vi "DBSCAN.vi"(8 "error in":errorcluster) -> (0 "error out":errorcluster, 3 "out":refnum<class "DBSCAN.lvclass">)   [LabVIEW 2020]
doc: "Perform DBSCAN clustering from vector array or distance matrix.\n\n DBSCAN - Density-Based Spatial Clustering of Applications with Noise.\n Finds core samples of high density and expands clusters from them.\n Good for data which contains clusters of similar density.\n\n Read more in the :ref:`User Guide <dbscan>`.\n\n Parameters\n ----------\n eps : float, default=0.5\n The maximum distance between two samples for one to be considered\n as in the neighborhood of the other. This is not a maximum bound\n on the distances of points within a cluster. This is the most\n important DBSCAN parameter to choose appropriately for your data set\n and distance function.\n\n min_samples : int, default=5\n The number of samples (or total weight) in a neighborhood for a point\n to be considered as a core point. This includes the point itself.\n\n metric : string, or callable, default='euclidean'\n The metric to use when calculating distance between instances in a\n feature array. If metric is a string or callable, it must be one of\n the options allowed by :func:`sklearn.metrics.pairwise_distances` for\n its metric parameter.\n If metric is \"precomputed\", X is assumed to be a distance matrix and\n must be square. X may be a :term:`Glossary <sparse graph>`, in which\n case only \"nonzero\" elements may be considered neighbors for DBSCAN.\n\n .. versionadded:: 0.17\n metric *precomputed* to accept precomputed sparse matrix.\n\n metric_params : dict, default=None\n Additional keyword arguments for the metric function.\n\n .. versionadded:: 0.19\n\n algorithm : {'auto', 'ball_tree', 'kd_tree', 'brute'}, default='auto'\n The algorithm to be used by the NearestNeighbors module\n to compute pointwise distances and find nearest neighbors.\n See NearestNeighbors module documentation for details.\n\n leaf_size : int, default=30\n Leaf size passed to BallTree or cKDTree. This can affect the speed\n of the construction and query, as well as the memory required\n to store the tree. The optimal value depends\n on the nature of the problem.\n\n p : float, default=None\n The power of the Minkowski metric to be used to calculate distance\n between points. If None, then ``p=2`` (equivalent to the Euclidean\n distance).\n\n n_jobs : int, default=None\n The number of parallel jobs to run.\n ``None`` means 1 unless in a :obj:`joblib.parallel_backend` context.\n ``-1`` means using all processors. See :term:`Glossary <n_jobs>`\n for more details.\n\n Attributes\n ----------\n core_sample_indices_ : ndarray of shape (n_core_samples,)\n Indices of core samples.\n\n components_ : ndarray of shape (n_core_samples, n_features)\n Copy of each core sample found by training.\n\n labels_ : ndarray of shape (n_samples)\n Cluster labels for each point in the dataset given to fit().\n Noisy samples are given the label -1.\n\n \nAvailable methods:\nGet Attributes\nGet Params\nSet Params"
uses:
  DBSCAN.lvclass
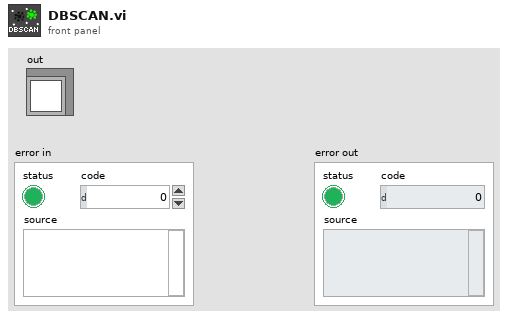
[diagram p1: front panel]
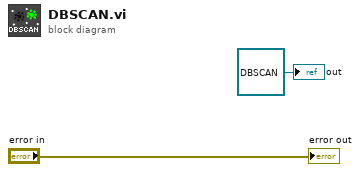
[diagram p0: block diagram]
diagram:
  "out" <- refnum<class "DBSCAN.lvclass"> refnum ("model")
  "error out" <- "error in"
